vi "CheckInheritance.vi"(8 "error in (no error)":errorcluster, 10 "Path":path, 11 "SMO.UI.MAUI in":refnum<class "SMO.UI.MAUI.lvclass">) -> (0 "error out":errorcluster, 1 "IsEmbedded?":bool, 2 "Path":path, 3 "SMO.UI.MAUI out":refnum<class "SMO.UI.MAUI.lvclass">)   [LabVIEW 2019, in "SMO.UI.MAUI.lvclass"]
uses:
  SMO.UI.MAUI.lvclass
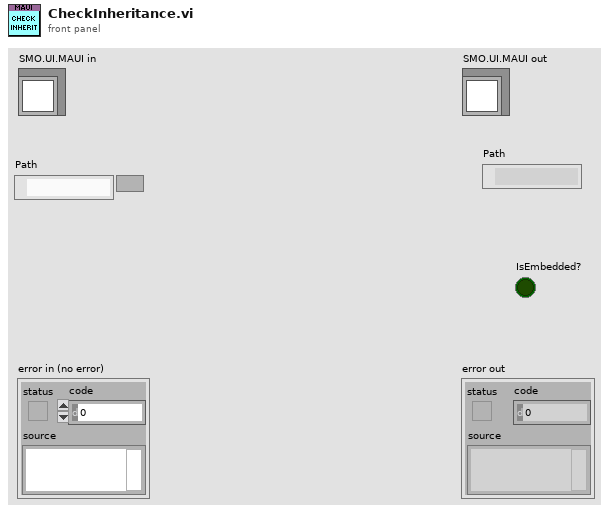
[diagram p1: front panel]
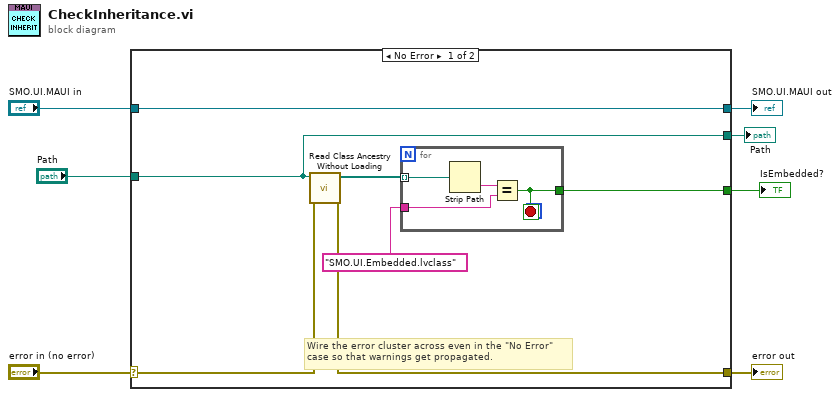
[diagram p0: block diagram]
diagram:
  n1 = case shown="No Error" "error in (no error)" {
    selector: "error in (no error)" -> [w13 w20]
    tunnel: [w12 w20] -> w6
    tunnel: [w14 w19] -> w4
    tunnel: "SMO.UI.MAUI in" -> [w14 w19]
    tunnel: "Path" -> [w8 _]
    tunnel: [w9 _] -> w2
    tunnel: [w8 _] -> w1
    frame No Error {
      # "Wire the error cluster across even in the \"No Error\"\ncase so that warnings get propagated."
      n2 = call <vilib>:"Read Class Ancestry Without Loading.vi"("error in (no error)"=w13, "LabVIEW Class Path"=w8) -> ("error out"=w12:errorcluster, "Class Ancestry"=w11:path[])  [unwired: 8 in]
      n3 = for {
        tunnel: w11 -> [w18] mode=indexing
        tunnel: [w15] -> w9
        tunnel: "SMO.UI.Embedded.lvclass" -> [w16]
        stop <- w15 stop-if-true
        n4 = Strip Path(path=w18) -> (name=w17:string)  [unwired: 1 out]
        n5 = Equal?(x=w17, y=w16) -> (x = y?=w15:bool)
      }
    }
    frame Error {
    }
  }
  "error out" <- w6
  "SMO.UI.MAUI out" <- w4
  "IsEmbedded?" <- w2
  "Path" <- w1
